vi "Average_Spectrum_XY.vi"(2 "Multiplyer":dbl, 3 "Array IN 3D":T1) -> (0 "Mean":dbl format="%0.2f", 1 "Array Out 1D":dbl[](array[numeric]))   [LabVIEW 2016]
uses:
  Control.ctl
  <vilib>/Analysis/baseanly.llb/Mean (DBL).vi
  <vilib>/Analysis/NI_AALBase.lvlib
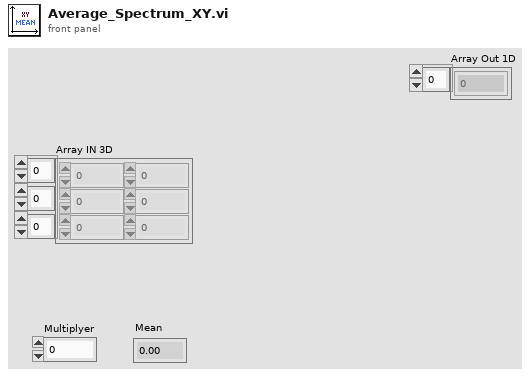
[diagram p1: front panel]
types:
  T1 = typedef "Control.ctl" = dbl[][][]
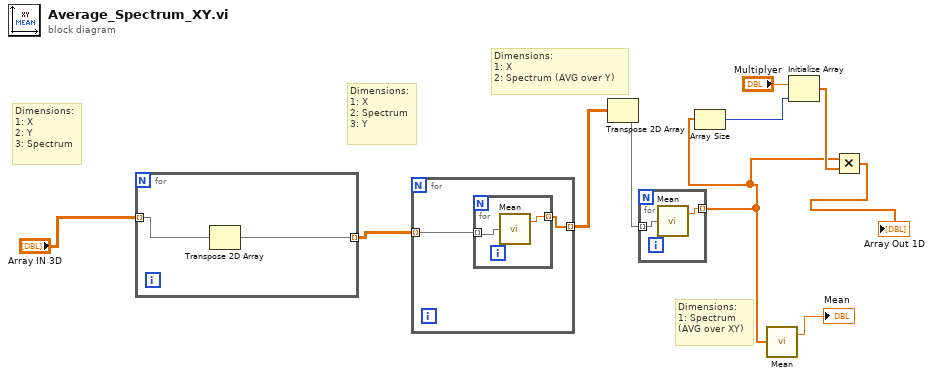
[diagram p0: block diagram]
diagram:
  # "Dimensions:\n1: Spectrum\n(AVG over XY)"
  # "Dimensions:\n1: X\n2: Spectrum (AVG over Y)"
  # "Dimensions:\n1: X\n2: Spectrum\n3: Y"
  # "Dimensions:\n1: X\n2: Y\n3: Spectrum"
  n1 = for {
    tunnel: "Array IN 3D" -> [w12] mode=indexing
    tunnel: [w11] -> w9 mode=indexing
    n2 = Transpose 2D Array(2D array=w12) -> (transposed array=w11:dbl[][])
  }
  n3 = for {
    tunnel: w9 -> [w14] mode=indexing
    tunnel: [w13] -> w8 mode=indexing
    n4 = for {
      tunnel: [w16] -> w13 mode=indexing
      tunnel: w14 -> [w15] mode=indexing
      n5 = call-poly <vilib>:"Mean.vi"("X"=w15) -> ("mean"=w16:dbl)  [unwired: 1 out]
    }
  }
  n6 = Transpose 2D Array(2D array=w8) -> (transposed array=w7:dbl[][])
  n7 = for {
    tunnel: [w18] -> w2 mode=indexing
    tunnel: w7 -> [w17] mode=indexing
    n8 = call-poly <vilib>:"Mean.vi"("X"=w17) -> ("mean"=w18:dbl)  [unwired: 1 out]
  }
  n9 = Array Size(array=w2) -> (size(s)=w5:i32)
  n10 = call-poly <vilib>:"Mean.vi"("X"=w2) -> ("mean"=→"Mean":dbl)  [unwired: 1 out]
  n11 = Initialize Array("Multiplyer", w5) -> (w6:dbl[])
  n12 = Multiply(x=w2, y=w6) -> (x*y=→"Array Out 1D":dbl[])
